vi "Write TSTRB Core.vi"(10 "value":bool[](array[boolean]), 11 "niInstr AXI4-Stream Writer v1 FPGA in":refnum<class "niInstr AXI4-Stream Writer v1 FPGA.lvclass">) -> (3 "niInstr AXI4-Stream Writer v1 FPGA out":refnum<class "niInstr AXI4-Stream Writer v1 FPGA.lvclass">)   [LabVIEW 2015, in "niInstr AXI4-Stream Writer v1 FPGA.lvclass"]
uses:
  <instrlib>/_niInstr/CLIP Adapters/v1/FPGA/AXI4-Stream/Writer/niInstr AXI4-Stream Writer v1 FPGA.lvclass
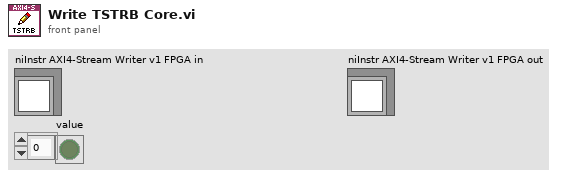
[diagram p1: front panel]
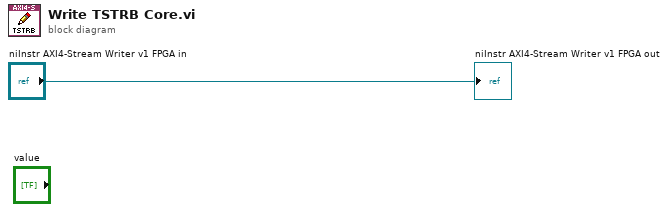
[diagram p0: block diagram]
diagram:
  "niInstr AXI4-Stream Writer v1 FPGA out" <- "niInstr AXI4-Stream Writer v1 FPGA in"
